vi "RT Communications Loop.vi"(9 "Comms data":T1={"Parameters"={"error writer name"="error writer", "command reader name"="command reader", "Host URL"="155.198.87.XXX", "error buffer size"=16, "command buffer size"=16}, "Variables"={"error stream"="", "comms stream"="", "listen schedule"=0}}, 11 "RT Queues":T2) -> ()   [LabVIEW 2018]
uses:
  Type Defs/Queues cluster.ctl
  Chris VIs/Message Scheduler/message scheduler.lvclass
  Communications loop/comms data.ctl
  Chris VIs/Incident logger/Incidents/Incident.lvclass
  Chris VIs/Incident logger/Incidents/Warning/Warning.lvclass
  Z:/OneDrive - Imperial College London/LabVIEW/Chris VIs/Incident logger/Incidents/Incident.lvclass
  Queue VIs/De-queue RT comms element.vi
  Queue VIs/En-queue RT comms element.vi
  Queue VIs/Close RT comms queue.vi
  Queue VIs/Queues.lvlib
  RT subVIs/Incident handling.lvlib
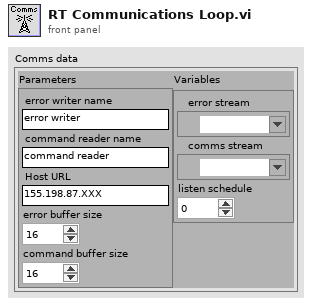
[diagram p1: front panel]
types:
  T1 = typedef "comms data.ctl" = cluster{"Parameters":cluster{"error writer name":string, "command reader name":string, "Host URL":string, "error buffer size":i32, "command buffer size":i32}, "Variables":cluster{"error stream":refnum<k21>, "comms stream":refnum<k21>, "listen schedule":u32}}
  T2 = typedef "Real-Time.lvlib/Queues.lvlib/Queues cluster.ctl" = cluster{"RT Message":refnum<queue>, "RT Comms":refnum<queue>, "RT Data":refnum<queue>, "message scheduler":refnum<class "message scheduler.lvclass">}
  T3 = cluster{"Target":string, "Loop":string, "Code":string}
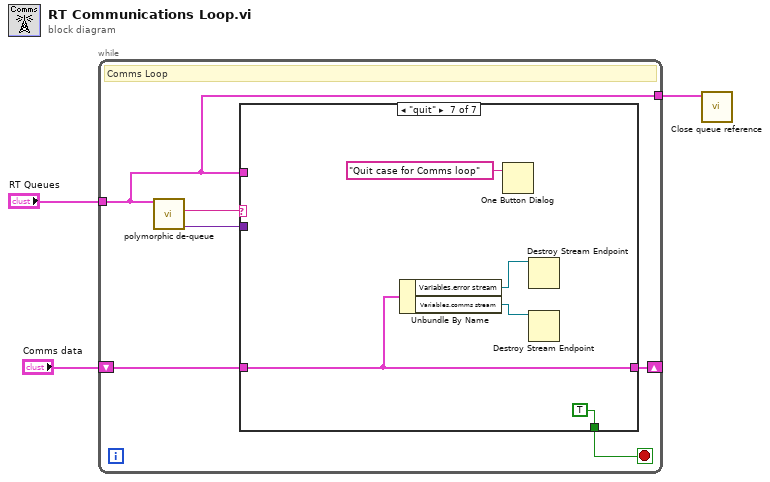
[diagram p0: block diagram]
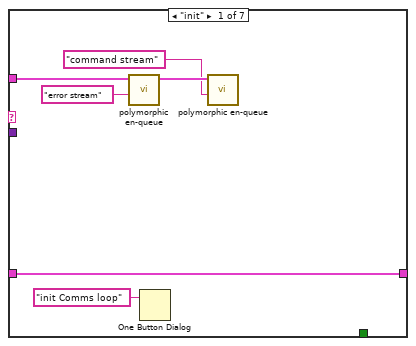
[diagram p2: hidden frame]
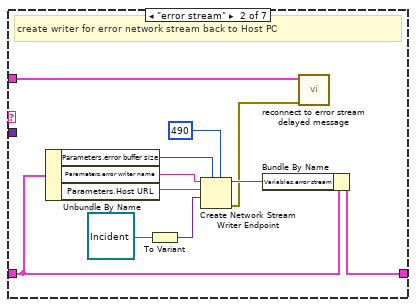
[diagram p3: hidden frame]
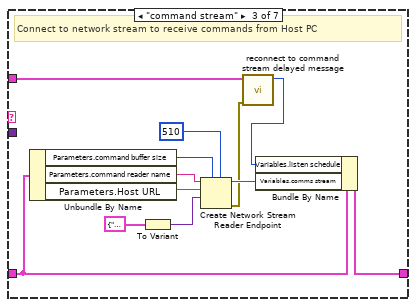
[diagram p4: hidden frame]
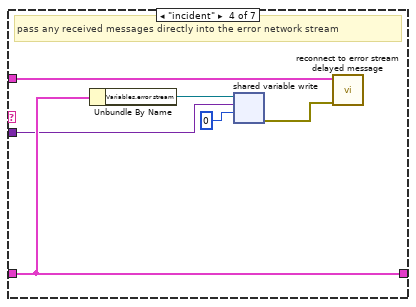
[diagram p5: hidden frame]
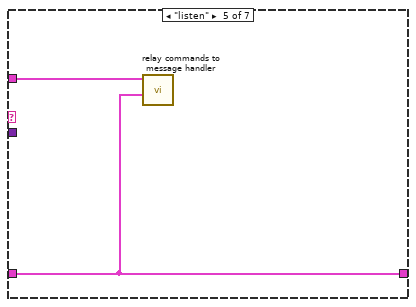
[diagram p6: hidden frame]
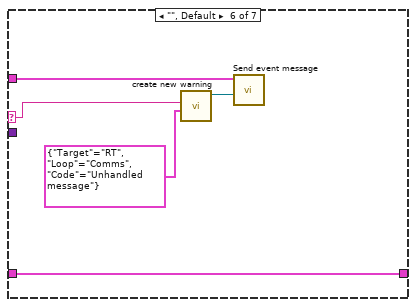
[diagram p7: hidden frame]
diagram:
  n1 = while {
    tunnel: "RT Queues" -> [w6]
    tunnel: [w6] -> w2
    shift-right: [w4] -> _
    shift-left: "Comms data" -> [w5]
    stop <- w7 stop-if-true
    # "Comms Loop"
    n2 = call-poly "polymorphic de-queue.vi"("RT Queues"=w6) -> ("Data"=w8:variant, "Message"=w9:string)  [unwired: 9 in]
    n3 = case shown="\"quit\"" w9 {
      selector: w9 -> [_ _ _ _ _ w50 _]
      tunnel: w8 -> [_ _ _ w42 _ _ _]
      tunnel: [_ _ _ _ _ _ TRUE] -> w7
      tunnel: w6 -> [w14 w16 w29 w39 w46 w51 _]
      tunnel: w5 -> [w10 w21 w34 w44 w45 w47 w52]
      tunnel: [w10 w20 w33 w44 w45 w47 w52] -> w4
      frame "init" {
        n4 = call-poly "polymorphic en-queue.vi"("Message"="error stream", "RT Queues"=w14) -> ("RT Queues out"=w12:T2)  [unwired: 9 in]
        n5 = One Button Dialog(message="init Comms loop") -> ()  [unwired: 1 in, 1 out]
        n6 = call-poly "polymorphic en-queue.vi"("Message"="command stream", "RT Queues"=w12) -> ()  [unwired: 9 in, 1 out]
      }
      frame "error stream" {
        # "create writer for error network stream back to Host PC"
        n7 = Unbundle By Name(w21) -> ("Parameters.error buffer size"=w22:i32, "Parameters.error writer name"=w24:string, "Parameters.Host URL"=w23:string)
        n8 = To Variant(anything=refnum<class "Incident.lvclass"> refnum ("incident logger.lvlib:Incident.lvclass")) -> (Variant=w26:variant)
        n9 = Create Network Stream Writer Endpoint(5:490 ("timeout in ms (-1)"), 7:w22, 9:w26, 10:w23, 11:w24) -> (0:w17:errorcluster, 3:w19:refnum<k21>)  [unwired: 2 in]
        n10 = Bundle By Name(cluster=w21, "Variables.error stream"=w19) -> (w20:T1)
        n11 = call "reconnect to error stream delayed message.vi"("error in (no error)"=w17, "RT Queues"=w16) -> ()  [unwired: 10 in]
      }
      frame "command stream" {
        # "Connect to network stream to receive commands from Host PC"
        n12 = Unbundle By Name(w34) -> ("Parameters.command buffer size"=w35:i32, "Parameters.command reader name"=w37:string, "Parameters.Host URL"=w36:string)
        n13 = To Variant(anything=cluster{"message":string, "data":variant} {"message"="", "data"=variant}) -> (Variant=w38:variant)
        n14 = Create Network Stream Reader Endpoint(5:510 ("timeout in ms (-1)"), 7:w35, 9:w38, 10:w36, 11:w37) -> (0:w28:errorcluster, 3:w31:refnum<k21>)  [unwired: 2 in]
        n15 = call "reconnect to command stream delayed message.vi"("error in (no error)"=w28, "RT Queues"=w29) -> ("schedule ID"=w27:u32)  [unwired: 9 in]
        n16 = Bundle By Name(cluster=w34, "Variables.listen schedule"=w27, "Variables.comms stream"=w31) -> (w33:T1)
      }
      frame "incident" {
        # "pass any received messages directly into the error network stream"
        n17 = Unbundle By Name(w44) -> ("Variables.error stream"=w43:refnum<k21>)
        n18 = shared-variable-write(w43, w42, 0 ("timeout ms (-1)")) -> (w40:errorcluster)  [unwired: 1 in, 2 out]
        n19 = call "reconnect to error stream delayed message.vi"("error in (no error)"=w40, "RT Queues"=w39) -> ()  [unwired: 10 in]
      }
      frame "listen" {
        n20 = call "relay commands to message handler.vi"("Comms data"=w45, "RT Queues"=w46) -> ()  [unwired: 10 in]
      }
      frame "", Default {
        n21 = call "create new warning.vi"("Location"=T3 {"Target"="RT", "Loop"="Comms", "Code"="Unhandled message"}, "Description"=w50) -> ("Warning out"=w48:refnum<class "Warning.lvclass">)  [unwired: 8 in, 1 out]
        n22 = call "Send event message.vi"("Incident"=w48, "RT Queues"=w51) -> ()  [unwired: 10 in]
      }
      frame "quit" {
        n23 = Unbundle By Name(w52) -> ("Variables.error stream"=w53:refnum<k21>, "Variables.comms stream"=w54:refnum<k21>)
        n24 = One Button Dialog(message="Quit case for Comms loop") -> ()  [unwired: 1 in, 1 out]
        n25 = Destroy Stream Endpoint(11:w53) -> ()  [unwired: 1 in, 1 out]
        n26 = Destroy Stream Endpoint(11:w54) -> ()  [unwired: 1 in, 1 out]
      }
    }
  }
  n27 = call-poly "Close queue reference.vi"("RT Queues"=w2) -> ()  [unwired: 11 in]
